vi "DoubleCoincidencesCheck.vi"(6 "Time B":dbl, 7 "Time A":dbl, 8 "ChB":dbl, 9 "ChA":dbl, 10 "Cluster In":T1 {"Coincidence Window" format="%#_13g"; "Delay12" format="%#_13g"; "Delay02" format="%#_13g"; "Delay01" format="%#_13g"}) -> (2 "cluster Out":T1 {"Coincidence Window" format="%#_13g"; "Delay12" format="%#_13g"; "Delay02" format="%#_13g"; "Delay01" format="%#_13g"})   [LabVIEW 2023]
uses:
  Get_Delays_Ctrl.ctl
panel:
  in  "Delays01 In":dbl[](array[numeric])
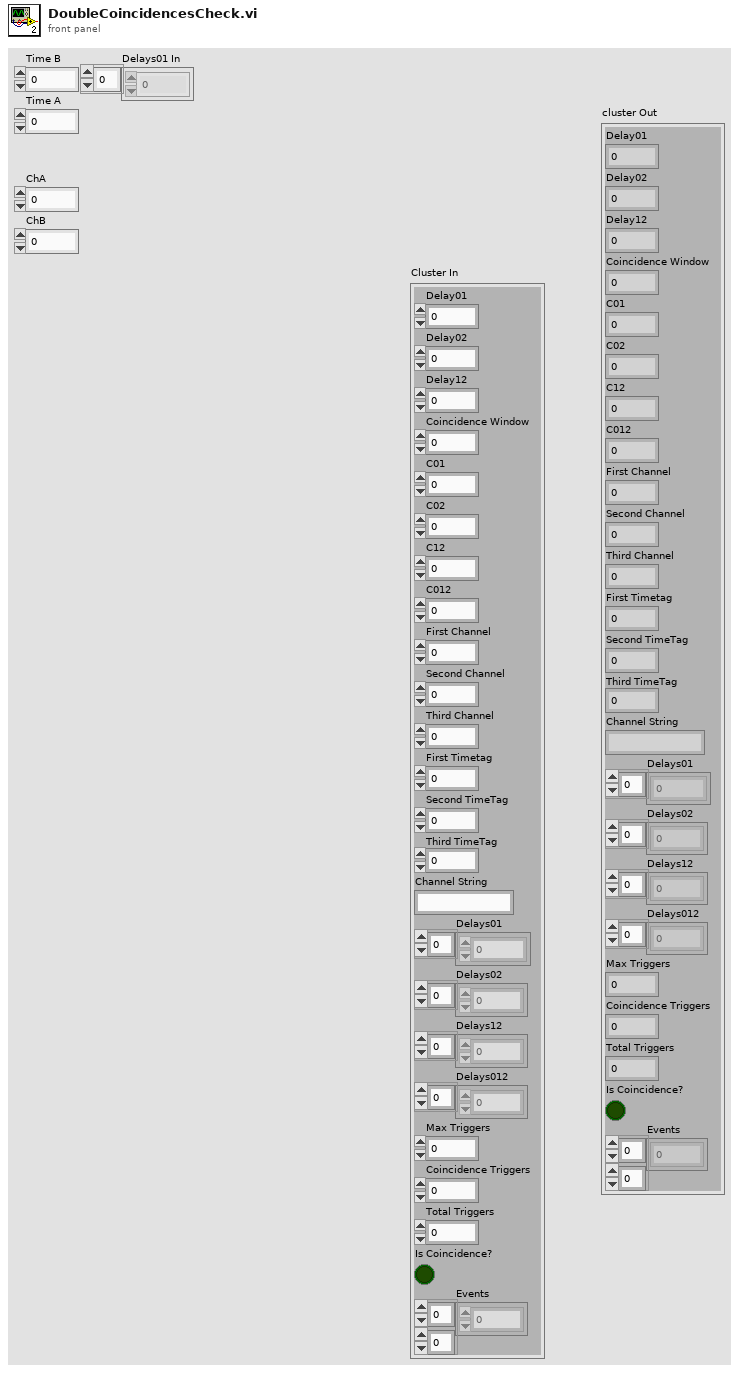
[diagram p1: front panel]
types:
  T1 = typedef "Get_Delays_Ctrl.ctl" = cluster{"Delay01":dbl, "Delay02":dbl, "Delay12":dbl, "Coincidence Window":dbl, "C01":u32, "C02":u32, "C12":u32, "C012":u32, "First Channel":dbl, "Second Channel":dbl, "Third Channel":dbl, "First Timetag":dbl, "Second TimeTag":dbl, "Third TimeTag":dbl, "Channel String":string, "Delays01":sgl[], "Delays02":dbl[], "Delays12":dbl[], "Delays012":dbl[], "Max Triggers":i32, "Coincidence Triggers":i32, "Total Triggers":i32, "Is Coincidence?":bool, "Events":u64[][]}
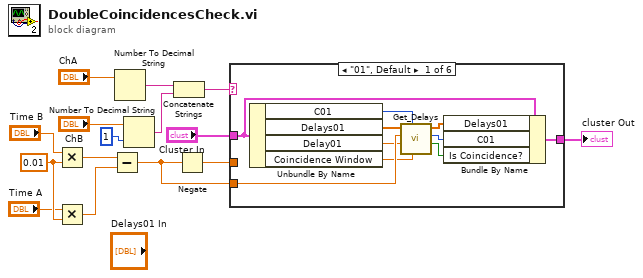
[diagram p0: block diagram]
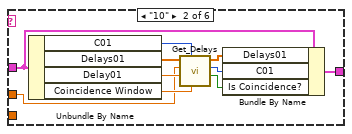
[diagram p2: hidden frame]
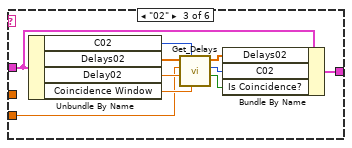
[diagram p3: hidden frame]
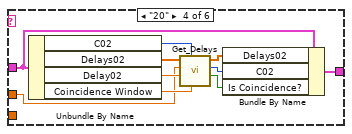
[diagram p4: hidden frame]
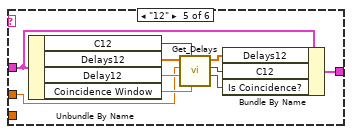
[diagram p5: hidden frame]
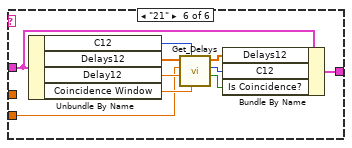
[diagram p6: hidden frame]
diagram:
  w12 = 0.01 ("y")
  n1 = Multiply(x="Time B", y=w12) -> (x*y=w7:dbl)
  n2 = Multiply(x="Time A", y=w12) -> (x*y=w8:dbl)
  n3 = Subtract(x=w7, y=w8) -> (x-y=w11:dbl)
  n4 = Number To Decimal String(number="ChA") -> (decimal integer string=w14:string)  [unwired: 1 in]
  n5 = Number To Decimal String(number="ChB", width (-)=i16 1) -> (decimal integer string=w15:string)
  n6 = Concatenate Strings(w14, w15) -> (w9:string)
  n7 = Negate(x=w11) -> (-x=w10:dbl)
  n8 = case shown="\"01\", Default" w9 {
    tunnel: w11 -> [w25 _ w37 _ _ w66]
    tunnel: w10 -> [_ w27 _ w46 w56 _]
    tunnel: "Cluster In" -> [w20 w31 w41 w51 w61 w71]
    tunnel: [w21 w32 w42 w52 w62 w72] -> w5
    frame "01", Default {
      n9 = Unbundle By Name(w20) -> ("C01"=w16:u32, "Delays01"=w19:sgl[], "Delay01"=w18:dbl, "Coincidence Window"=w17:dbl)
      n10 = call "Get_Delays.vi"("Coincidence Window"=w17, "Coincidences In"=w16, "Expected Delay"=w18, "Delay"=w25, "Delays In"=w19) -> ("Is Coincidence?"=w22:bool, "Coincidences out"=w23:u32, "Delays Out"=w24:dbl[])  [unwired: 4 in]
      n11 = Bundle By Name(cluster=w20, "Delays01"=w24, "C01"=w23, "Is Coincidence?"=w22) -> (w21:T1)
    }
    frame "10" {
      n12 = Unbundle By Name(w31) -> ("C01"=w26:u32, "Delays01"=w30:sgl[], "Delay01"=w29:dbl, "Coincidence Window"=w28:dbl)
      n13 = call "Get_Delays.vi"("Coincidence Window"=w28, "Coincidences In"=w26, "Expected Delay"=w29, "Delay"=w27, "Delays In"=w30) -> ("Is Coincidence?"=w33:bool, "Coincidences out"=w34:u32, "Delays Out"=w35:dbl[])  [unwired: 4 in]
      n14 = Bundle By Name(cluster=w31, "Delays01"=w35, "C01"=w34, "Is Coincidence?"=w33) -> (w32:T1)
    }
    frame "02" {
      n15 = Unbundle By Name(w41) -> ("C02"=w36:u32, "Delays02"=w40:dbl[], "Delay02"=w38:dbl, "Coincidence Window"=w39:dbl)
      n16 = call "Get_Delays.vi"("Coincidence Window"=w39, "Coincidences In"=w36, "Expected Delay"=w38, "Delay"=w37, "Delays In"=w40) -> ("Is Coincidence?"=w43:bool, "Coincidences out"=w44:u32, "Delays Out"=w45:dbl[])  [unwired: 4 in]
      n17 = Bundle By Name(cluster=w41, "Delays02"=w45, "C02"=w44, "Is Coincidence?"=w43) -> (w42:T1)
    }
    frame "20" {
      n18 = Unbundle By Name(w51) -> ("C02"=w47:u32, "Delays02"=w50:dbl[], "Delay02"=w48:dbl, "Coincidence Window"=w49:dbl)
      n19 = call "Get_Delays.vi"("Coincidence Window"=w49, "Coincidences In"=w47, "Expected Delay"=w48, "Delay"=w46, "Delays In"=w50) -> ("Is Coincidence?"=w53:bool, "Coincidences out"=w54:u32, "Delays Out"=w55:dbl[])  [unwired: 4 in]
      n20 = Bundle By Name(cluster=w51, "Delays02"=w55, "C02"=w54, "Is Coincidence?"=w53) -> (w52:T1)
    }
    frame "12" {
      n21 = Unbundle By Name(w61) -> ("C12"=w57:u32, "Delays12"=w60:dbl[], "Delay12"=w58:dbl, "Coincidence Window"=w59:dbl)
      n22 = call "Get_Delays.vi"("Coincidence Window"=w59, "Coincidences In"=w57, "Expected Delay"=w58, "Delay"=w56, "Delays In"=w60) -> ("Is Coincidence?"=w63:bool, "Coincidences out"=w64:u32, "Delays Out"=w65:dbl[])  [unwired: 4 in]
      n23 = Bundle By Name(cluster=w61, "Delays12"=w65, "C12"=w64, "Is Coincidence?"=w63) -> (w62:T1)
    }
    frame "21" {
      n24 = Unbundle By Name(w71) -> ("C12"=w67:u32, "Delays12"=w70:dbl[], "Delay12"=w68:dbl, "Coincidence Window"=w69:dbl)
      n25 = call "Get_Delays.vi"("Coincidence Window"=w69, "Coincidences In"=w67, "Expected Delay"=w68, "Delay"=w66, "Delays In"=w70) -> ("Is Coincidence?"=w73:bool, "Coincidences out"=w74:u32, "Delays Out"=w75:dbl[])  [unwired: 4 in]
      n26 = Bundle By Name(cluster=w71, "Delays12"=w75, "C12"=w74, "Is Coincidence?"=w73) -> (w72:T1)
    }
  }
  "cluster Out" <- w5
